vi "TIO Data Stream Convert.vi"(11 "Data Stream Notification":T1={"Stream Description"={"Stream ID"=0, "Data Type"=66, "Channels"=3, "Restart ID"=0, "Start timestamp (s)"=0.20090000000000002, "Sample counter"=382825, "Period (s)"=0.005, "Flags"=1, "Timestamp type"=1, "Name"="gmr.cal", "Last sample number"=0, "Last Restart ID"=0, "Version"=0, "Sample Size"=0}, "Sample #"=0, "Raw Data"=""} {"Stream Description"."Timestamp type" format="%x"; "Stream Description"."Flags" format="%x"; "Stream Description"."Data Type" items=["INT8"=16, "UINT8"=17, "UINT16"=32, "INT16"=33, "UINT24"=48, "INT24"=49, "UINT32"=64, "INT32"=65, "UINT64"=128, "INT64"=129, "FLOAT32"=66, "FLOAT64"=130]}) -> (3 "Waveform":cluster{dbl, dbl, dbl[][]})   [LabVIEW 2016]
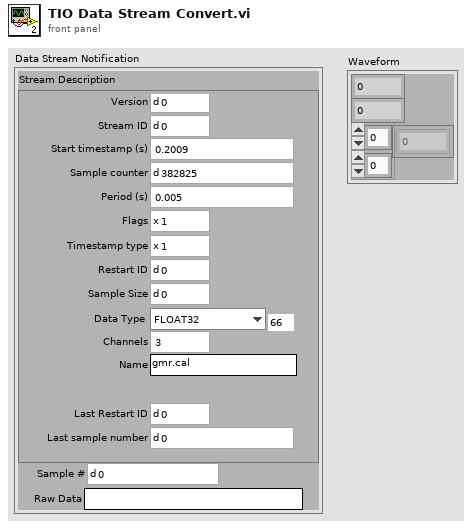
[diagram p1: front panel]
types:
  T1 = cluster{"Stream Description":cluster{"Stream ID":u16, "Data Type":u8, "Channels":u8, "Restart ID":u16, "Start timestamp (s)":dbl, "Sample counter":u64, "Period (s)":dbl, "Flags":u8, "Timestamp type":u8, "Name":string, "Last sample number":u64, "Last Restart ID":u16, "Version":u16, "Sample Size":u16}, "Sample #":u32, "Raw Data":string}
  T2 = enum16{"big-endian, network order", "native, host order", "little-endian"}
  T3 = cluster{"Stream ID":u16, "Data Type":u8, "Channels":u8, "Restart ID":u16, "Start timestamp (s)":dbl, "Sample counter":u64, "Period (s)":dbl, "Flags":u8, "Timestamp type":u8, "Name":string, "Last sample number":u64, "Last Restart ID":u16, "Version":u16, "Sample Size":u16}
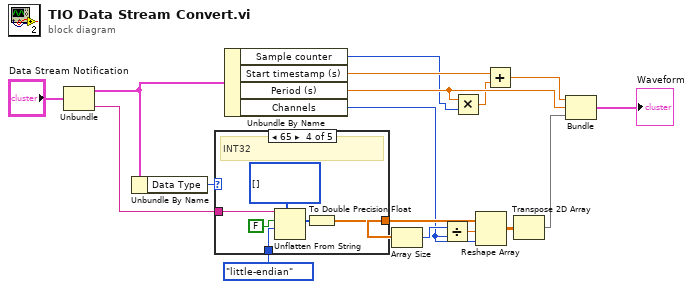
[diagram p0: block diagram]
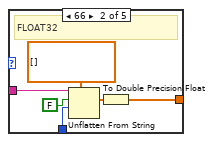
[diagram p3: hidden frame]
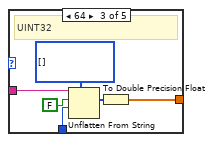
[diagram p4: hidden frame]
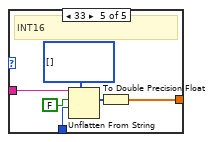
[diagram p5: hidden frame]
diagram:
  n1 = Unbundle("Data Stream Notification") -> ("Stream Description"=w14:T3, "Raw Data"=w16:string)  [unwired: 1 out]
  n2 = Unbundle By Name(w14) -> ("Data Type"=w15:u8)
  n3 = case shown="65" w15 {
    tunnel: w16 -> [_ w22 w28 w34 w40]
    tunnel: [_ w20 w26 w32 w38] -> w10
    tunnel: T2."little-endian" ("byte order (0:big-endian, network order)") -> [_ w18 w24 w30 w36]
    frame Default {
    }
    frame 66 {
      # "FLOAT32"
      n4 = Unflatten From String(type=sgl[] [], binary string=w22, data includes array or string size? (T)=FALSE, byte order (0:big-endian, network order)=w18) -> (value=w21:sgl[])  [unwired: 1 in, 2 out]
      n5 = To Double Precision Float(number=w21) -> (double precision float=w20:dbl[])
    }
    frame 64 {
      # "UINT32"
      n6 = Unflatten From String(type=u32[] [], binary string=w28, data includes array or string size? (T)=FALSE, byte order (0:big-endian, network order)=w24) -> (value=w27:u32[])  [unwired: 1 in, 2 out]
      n7 = To Double Precision Float(number=w27) -> (double precision float=w26:dbl[])
    }
    frame 65 {
      # "INT32"
      n8 = Unflatten From String(type=i32[] [], binary string=w34, data includes array or string size? (T)=FALSE, byte order (0:big-endian, network order)=w30) -> (value=w33:i32[])  [unwired: 1 in, 2 out]
      n9 = To Double Precision Float(number=w33) -> (double precision float=w32:dbl[])
    }
    frame 33 {
      # "INT16"
      n10 = Unflatten From String(type=i16[] [], binary string=w40, data includes array or string size? (T)=FALSE, byte order (0:big-endian, network order)=w36) -> (value=w39:i16[])  [unwired: 1 in, 2 out]
      n11 = To Double Precision Float(number=w39) -> (double precision float=w38:dbl[])
    }
  }
  n12 = Unbundle By Name(w14) -> ("Sample counter"=w1:u64, "Start timestamp (s)"=w3:dbl, "Period (s)"=w5:dbl, "Channels"=w7:u8)
  n13 = Array Size(array=w10) -> (size(s)=w9:i32)
  n14 = Divide(x=w9, y=w7) -> (x/y=w8:dbl)
  n15 = Multiply(x=w5, y=w1) -> (x*y=w4:dbl)
  n16 = Reshape Array(w10, w8, w7) -> (w12:dbl[][])
  n17 = Add(x=w3, y=w4) -> (x+y=w2:dbl)
  n18 = Transpose 2D Array(2D array=w12) -> (transposed array=w11:dbl[][])
  n19 = Bundle(w2, "Period (s)"=w5, w11) -> (→"Waveform":cluster{dbl, "Period (s)":dbl, dbl[][]})  [unwired: 1 in]
